vi "Prepare BMI Classification.vi"() -> (1 "Testing Array":dbl[][](array[numeric]), 2 "Teaching Set":T1[](array[typedef]), 3 "Classification":refnum<class "3D Plot Datatype.lvclass">[](array[class]))   [LabVIEW 2011, in "Super Simple Neural Network.lvlib"]
uses:
  Super Simple Neural Network.lvlib
  Types/1D Array.ctl
  Types/Teaching Vector.ctl
  <vilib>/Math Plots/3D Math Plots/3D Scatter/3D Scatter Datatype/3D Scatter Datatype.lvclass
  <vilib>/Math Plots/3D Math Plots/3D Scatter/3D Scatter Datatype/Public/Plot Helper (Vector).vi
  <vilib>/Math Plots/3D Math Plots/3D Plot/3D Plot Datatype/3D Plot Datatype.lvclass
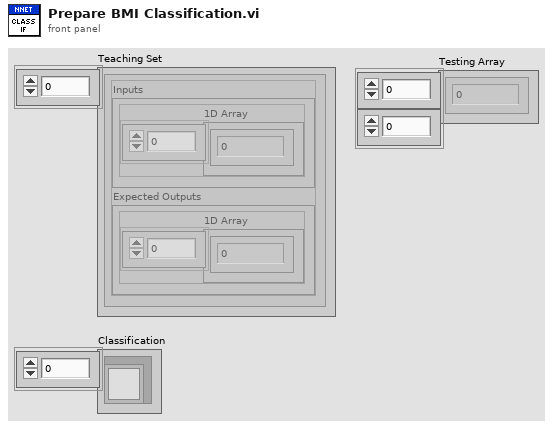
[diagram p1: front panel]
types:
  T1 = typedef "Super Simple Neural Network.lvlib/Teaching Vector.ctl" = cluster{"Inputs":T2, "Expected Outputs":T2}
  T2 = typedef "Super Simple Neural Network.lvlib/1D Array.ctl" = cluster{"1D Array":dbl[]}
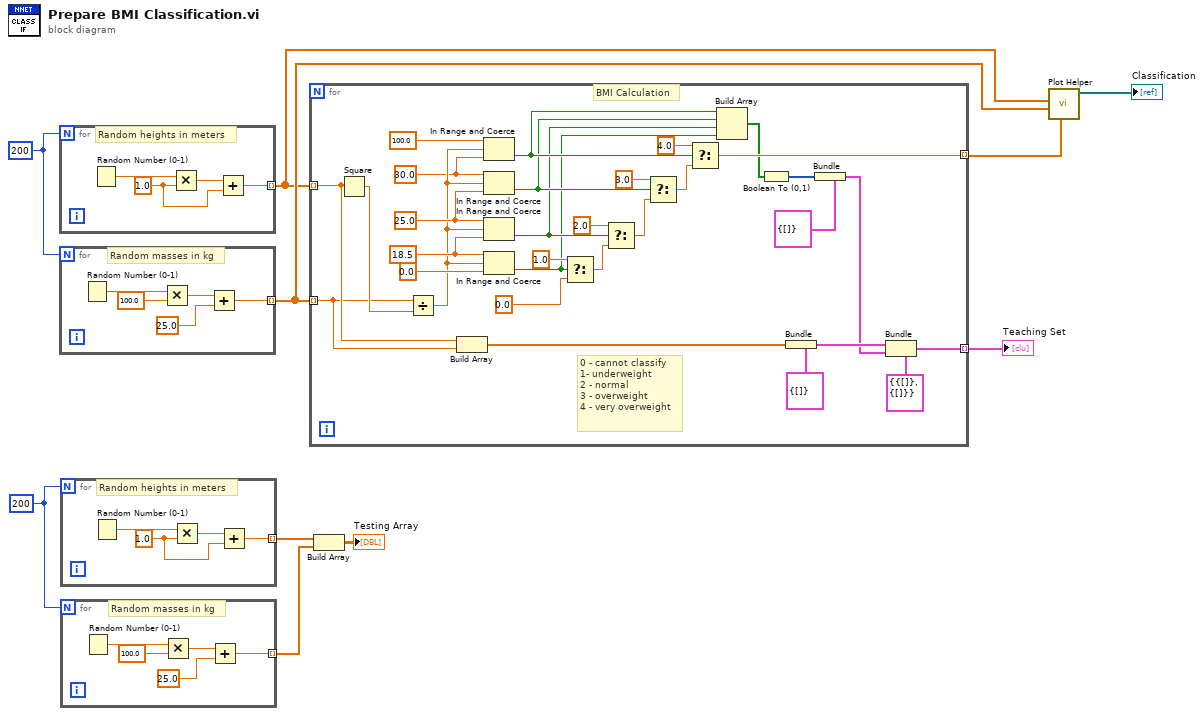
[diagram p0: block diagram]
diagram:
  w4 = 200
  w5 = 200
  n1 = for {
    N: w5 -> [_]
    tunnel: [w11] -> w7 mode=indexing
    w12 = 1.0 ("y")
    # "Random heights in meters"
    n2 = Random Number (0-1)() -> (number: 0 to 1=w14:dbl)
    n3 = Multiply(x=w14, y=w12) -> (x*y=w13:dbl)
    n4 = Add(x=w13, y=w12) -> (x+y=w11:dbl)
  }
  n5 = for {
    N: w5 -> [_]
    tunnel: [w15] -> w8 mode=indexing
    # "Random masses in kg"
    n6 = Random Number (0-1)() -> (number: 0 to 1=w17:dbl)
    n7 = Multiply(x=w17, y=100.0) -> (x*y=w18:dbl)
    n8 = Add(x=w18, y=25.0) -> (x+y=w15:dbl)
  }
  n9 = for {
    N: w4 -> [_]
    tunnel: [w20] -> w3 mode=indexing
    w21 = 1.0 ("y")
    # "Random heights in meters"
    n10 = Random Number (0-1)() -> (number: 0 to 1=w23:dbl)
    n11 = Multiply(x=w23, y=w21) -> (x*y=w22:dbl)
    n12 = Add(x=w22, y=w21) -> (x+y=w20:dbl)
  }
  n13 = for {
    N: w4 -> [_]
    tunnel: [w24] -> w2 mode=indexing
    # "Random masses in kg"
    n14 = Random Number (0-1)() -> (number: 0 to 1=w26:dbl)
    n15 = Multiply(x=w26, y=100.0) -> (x*y=w27:dbl)
    n16 = Add(x=w27, y=25.0) -> (x+y=w24:dbl)
  }
  n17 = for {
    tunnel: w7 -> [w45] mode=indexing
    tunnel: w8 -> [w44] mode=indexing
    tunnel: [w41] -> w9 mode=indexing
    tunnel: [w38] -> w10 mode=indexing
    w54 = 30.0 ("upper limit")
    w56 = 25.0 ("upper limit")
    w57 = 18.5 ("upper limit")
    # "0 - cannot classify\n1- underweight\n2 - normal\n3 - overweight\n4 - very overweight"
    # "BMI Calculation"
    n18 = Square(x=w45) -> (x^2=w59:dbl)
    n19 = Divide(x=w44, y=w59) -> (x/y=w55:dbl)
    n20 = Build Array(w45, w44) -> (w37:dbl[])
    n21 = In Range and Coerce(upper limit=100.0, x=w55, lower limit=w54) -> (In Range?=w34:bool)  [unwired: 1 out]
    n22 = In Range and Coerce(upper limit=w54, x=w55, lower limit=w56) -> (In Range?=w33:bool)  [unwired: 1 out]
    n23 = In Range and Coerce(upper limit=w56, x=w55, lower limit=w57) -> (In Range?=w32:bool)  [unwired: 1 out]
    n24 = In Range and Coerce(upper limit=w57, x=w55, lower limit=0.0) -> (In Range?=w31:bool)  [unwired: 1 out]
    n25 = Select(t=1.0, s=w31, f=0.0) -> (s? t:f=w48:dbl)
    n26 = Select(t=2.0, s=w32, f=w48) -> (s? t:f=w47:dbl)
    n27 = Select(t=3.0, s=w33, f=w47) -> (s? t:f=w46:dbl)
    n28 = Select(t=4.0, s=w34, f=w46) -> (s? t:f=w41:dbl)
    n29 = Build Array(w34, w33, w32, w31) -> (w30:bool[])
    n30 = Boolean To (0,1)(Boolean=w30) -> (0, 1=w29:i16[])
    n31 = Bundle(cluster=T2 {"1D Array"=[]} ("Inputs"), "1D Array"=w37) -> (w36:T2)
    n32 = Bundle(cluster=T2 {"1D Array"=[]} ("Expected Outputs"), "1D Array"=w29) -> (w35:T2)
    n33 = Bundle(cluster=T1 {"Inputs"={"1D Array"=[]}, "Expected Outputs"={"1D Array"=[]}}, "Inputs"=w36, "Expected Outputs"=w35) -> (w38:T1)
  }
  "Teaching Set" <- w10
  n34 = Build Array(w3, w2) -> (→"Testing Array":dbl[][])
  n35 = call-poly <vilib>:"Plot Helper.vi"("z vector"=w9, "y vector"=w8, "x vector"=w7) -> ("3D Plot lvclass Array out"=→"Classification":refnum<class "3D Plot Datatype.lvclass">[])  [unwired: 3 in, 5 out]
